vi "Fail.vi"(8 "error in (no error)":errorcluster, 9 "Message (\"\")":string, 10 "Actual":variant, 11 "Constraint in":refnum<class "Constraint.lvclass">) -> (0 "error out":errorcluster, 3 "Constraint out":refnum<class "Constraint.lvclass">)   [LabVIEW 2017, in "Transparent Assertions.lvlib" / "Constraints.lvlib" / "Constraint.lvclass"]
doc: "Generates an error for the given value. Optionally adds a message."
uses:
  Constraint.lvclass
  Frameworks/Test Framework/Test Framework.lvclass
  Frameworks/Test Framework Factory/Test Framework Factory.lvclass
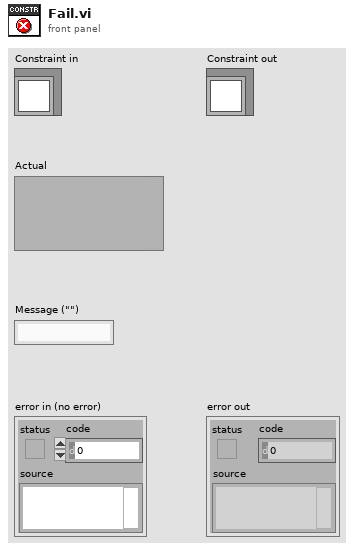
[diagram p1: front panel]
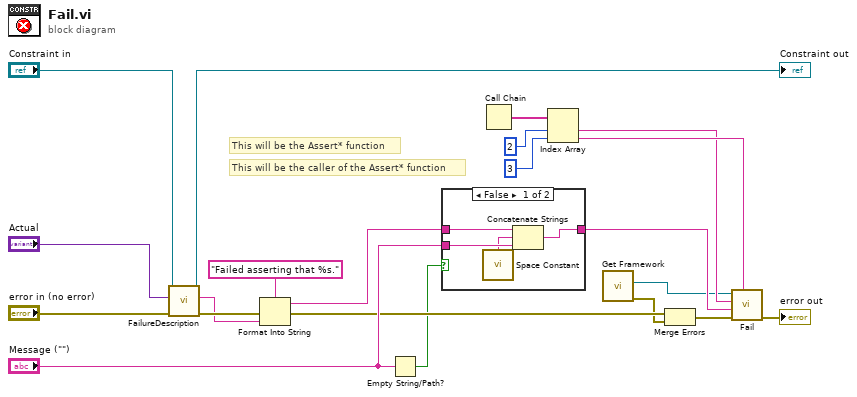
[diagram p0: block diagram]
diagram:
  # "This will be the Assert* function"
  # "This will be the caller of the Assert* function"
  n1 = call-dynamic "FailureDescription.vi"("error in (no error)"="error in (no error)", "Actual"="Actual", "Constraint in"="Constraint in") -> ("error out"=w13:errorcluster, "Failure Description"=w12:string, "Constraint out"=→"Constraint out":refnum<class "Constraint.lvclass">)  [unwired: 6 in]
  n2 = Format Into String(format string="Failed asserting that %s.", error in=w13, w12) -> (resulting string=w11:string, error out=w14:errorcluster)  [unwired: 1 in]
  n3 = Empty String/Path?(string/path="Message (\"\")") -> (empty?=w10:bool)
  n4 = case shown="False" w10 {
    tunnel: "Message (\"\")" -> [w25 _]
    tunnel: w11 -> [w23 w26]
    tunnel: [w22 w26] -> w9
    frame False {
      n5 = call <vilib>:"Space Constant.vi"() -> ("String"=w24:string)
      n6 = Concatenate Strings(w23, w24, w25) -> (w22:string)
    }
    frame True {
    }
  }
  n7 = Call Chain() -> (call chain=w8:string[])
  n8 = Index Array(array=w8, index #1=2 ("index"), index #2=3 ("index")) -> (element #1=w4:string, element #2=w7:string)
  n9 = call "Get Framework.vi"() -> ("error out"=w1:errorcluster, "Test Framework"=w3:refnum<class "Test Framework.lvclass">)  [unwired: 10 in]
  n10 = Merge Errors(w14, w1) -> (w2:errorcluster)
  n11 = call-dynamic "Fail.vi"("Caller"=w7, "error in (no error)"=w2, "Message"=w9, "Assertion"=w4, "Test Framework in"=w3) -> ("error out"=→"error out":errorcluster)  [unwired: 5 in, 1 out]
